vi "I2C_Send_7_Bit_Address_DAQ.vi"(1 "Write or Read?":bool, 2 "Receiver_7_Bit_Address":u8 format="%02x") -> ()   [LabVIEW 2022 SP3]
doc: "Petrus Prins 7 June 2026"
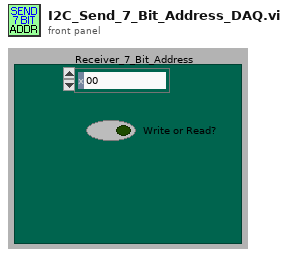
[diagram p1: front panel]
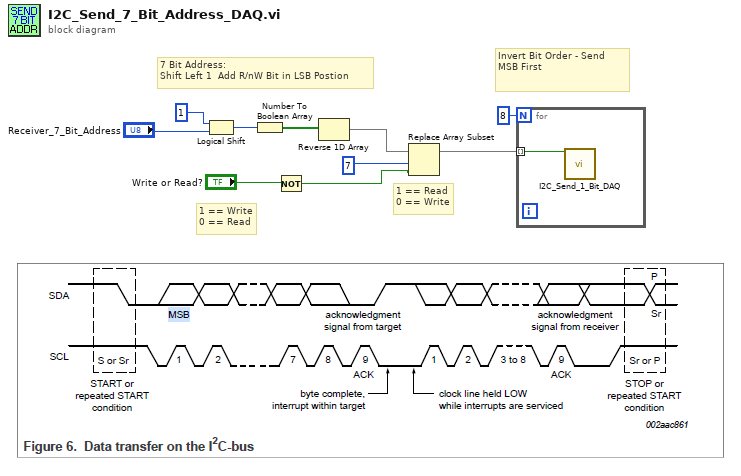
[diagram p0: block diagram]
diagram:
  # "1 == Write\n0 == Read"
  # "1 == Read\n0 == Write"
  # "Invert Bit Order - Send MSB First"
  # "7 Bit Address:\nShift Left 1  Add R/nW Bit in LSB Postion"
  n1 = Logical Shift(y=u8 1 ("x"), x="Receiver_7_Bit_Address") -> (x << y=w5:u8)
  n2 = Number To Boolean Array(number=w5) -> (Boolean array=w9:bool[])
  n3 = Not(x="Write or Read?") -> (.not. x?=w1:bool)
  n4 = Reverse 1D Array(array=w9) -> (reversed array=w8:bool[])
  n5 = Replace Array Subset(array=w8, new element=w1, index=7) -> (w6:bool[])
  n6 = for {
    N: 8 -> [_]
    tunnel: w6 -> [w11] mode=indexing
    n7 = call "I2C_Send_1_Bit_DAQ.vi"("Data_Bit"=w11) -> ()  [unwired: 2 in]
  }
